vi "Numeric Array to String.vi"(10 "List Data":dbl[](array[numeric])) -> (2 "Result String":string)   [LabVIEW 2026, in "Agilent B2900 Series.lvlib"]
doc: "Parse a numeric array into a comma separated string which can be recognized by SCPI commands"
uses:
  Agilent B2900 Series.lvlib
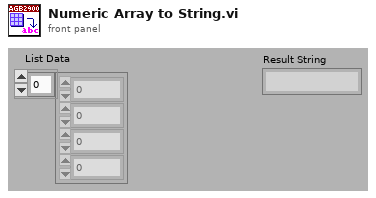
[diagram p1: front panel]
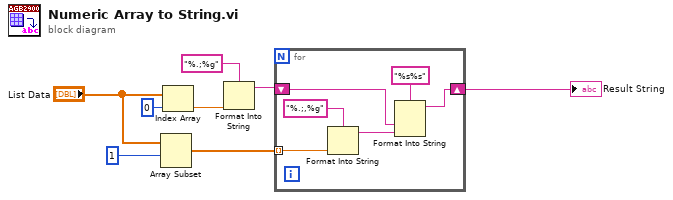
[diagram p0: block diagram]
diagram:
  n1 = Array Subset(array="List Data", index=1) -> (w7:dbl[])  [unwired: 1 in]
  n2 = Index Array(array="List Data", index=0) -> (element=w2:dbl)
  n3 = Format Into String(format string="%.;%g", w2) -> (resulting string=w1:string)  [unwired: 2 in, 1 out]
  n4 = for {
    tunnel: w7 -> [w14] mode=indexing
    shift-right: [w12] -> w8
    shift-left: w1 -> [w11]
    n5 = Format Into String(format string="%.;,%g", w14) -> (resulting string=w10:string)  [unwired: 2 in, 1 out]
    n6 = Format Into String(format string="%s%s", w11, w10) -> (resulting string=w12:string)  [unwired: 2 in, 1 out]
  }
  "Result String" <- w8
